vi "LV Test Semaphore 2.vi"() -> ()   [LabVIEW 2011]
panel:
  in  "milliseconds to wait":u32=500
  out "Wait Time":u32
  out "Hold Time":u32
  out "millisecond timer value 1":u32
  out "millisecond timer value 2":u32
  out "Locked 1":bool
  out "Numeric":i32
  out "Timed Out? 1":bool
  out "error out rel 2":errorcluster
  out "error out acq 2":errorcluster
  in  "Acq":bool
  in  "Open":bool
  in  "stop":bool
  out "Handle":u16
  out "error out create":errorcluster
  in  "Name":string="LabVIEW_System_Semaphore"
  out "error out destroy 1":errorcluster
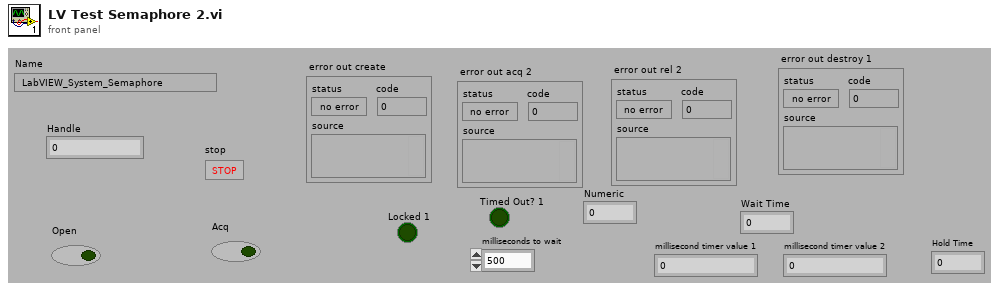
[diagram p1: front panel]
types:
  T1 = typedef "Semaphore RefNum" = refnum<k1>
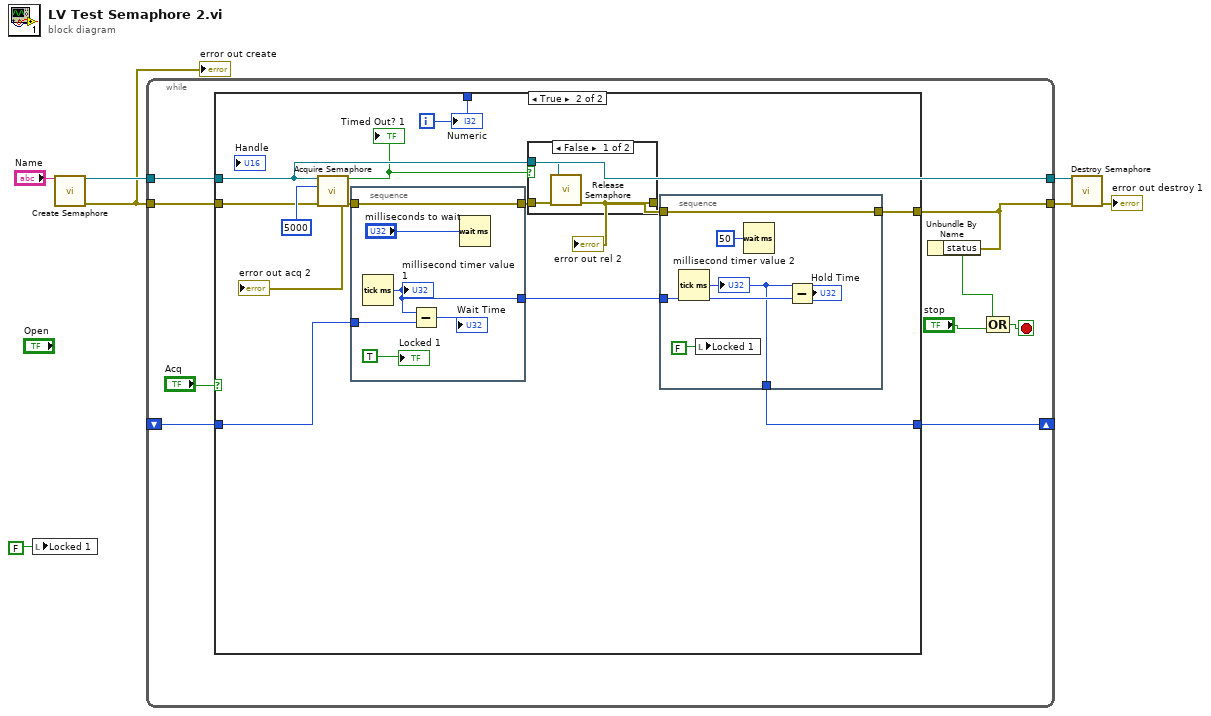
[diagram p0: block diagram]
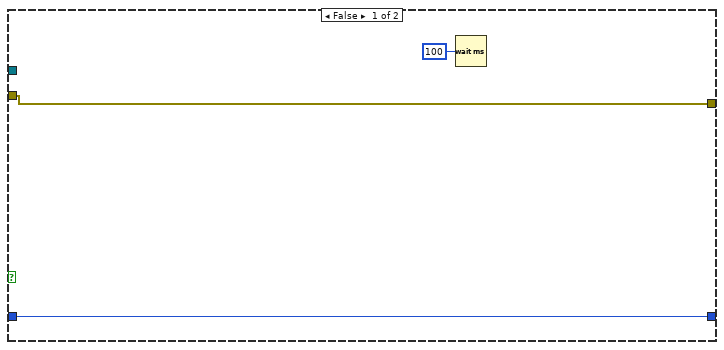
[diagram p2: hidden frame]
diagram:
  n1 = local write "Locked 1"(FALSE) -> ()
  n2 = call <vilib>:"Create Semaphore.vi"("name (unnamed)"="Name") -> ("error out"=w2:errorcluster, "semaphore"=w7:T1)  [unwired: 2 in, 3 out]
  "error out create" <- w2
  n3 = while {
    tunnel: w2 -> [w10]
    tunnel: w7 -> [w13]
    tunnel: [w13] -> w6
    tunnel: [w12] -> w5
    shift-right: [w9] -> _
    shift-left: _ -> [w8]
    i -> [w14]
    stop <- w16 stop-if-true
    n4 = case shown="True" "Acq" {
      tunnel: w14 -> [_ w32]
      tunnel: w13 -> [_ w26]
      tunnel: [w20 w30] -> w12
      tunnel: w10 -> [w20 w25]
      tunnel: [w18 w23] -> w9
      tunnel: w8 -> [w18 w22]
      frame False {
        n5 = Wait (ms)(milliseconds to wait=u32 100) -> ()  [unwired: 1 out]
      }
      frame True {
        n6 = call <vilib>:"Acquire Semaphore.vi"("error in (no error)"=w25, "ms timeout (-1)"=u16 5000 ("Timeout (ms)"), "semaphore"=w26) -> ("error out"=w29:errorcluster, "timed out"=w21:bool)  [unwired: 3 out]
        "Timed Out? 1" <- w21
        "error out acq 2" <- w29
        n7 = stacked-sequence {
          tunnel: w29 -> [w48]
          tunnel: [w48] -> w28
          tunnel: [w45] -> w24
          tunnel: w22 -> [w44]
          frame #0 {
            n8 = Tick Count (ms)() -> (millisecond timer value=w45:u32)
            "millisecond timer value 1" <- w45
            n9 = Subtract(x=w45, y=w44) -> (x-y=→"Wait Time":u32)
            n10 = Wait (ms)(milliseconds to wait="milliseconds to wait") -> ()  [unwired: 1 out]
            "Locked 1" <- TRUE
          }
        }
        n11 = case shown="False" w21 {
          tunnel: w28 -> [w35 w36]
          tunnel: w26 -> [w34 _]
          tunnel: [w33 w36] -> w27
          frame False {
            n12 = call <vilib>:"Release Semaphore.vi"("error in (no error)"=w35, "semaphore"=w34) -> ("error out"=w33:errorcluster)  [unwired: 5 out]
          }
          frame True {
          }
        }
        "error out rel 2" <- w27
        n13 = stacked-sequence {
          tunnel: w27 -> [w42]
          tunnel: [w42] -> w30
          tunnel: w24 -> [w39]
          tunnel: [w37] -> w23
          frame #0 {
            n14 = Tick Count (ms)() -> (millisecond timer value=w37:u32)
            "millisecond timer value 2" <- w37
            n15 = local write "Locked 1"(FALSE) -> ()
            n16 = Wait (ms)(milliseconds to wait=u32 50) -> ()  [unwired: 1 out]
            n17 = Subtract(x=w37, y=w39) -> (x-y=→"Hold Time":u32)
          }
        }
        "Numeric" <- w32
      }
    }
    n18 = Unbundle By Name(w12) -> ("status"=w15:bool)
    n19 = Compound Arithmetic op=OR(w15, "stop") -> (w16:bool)
  }
  n20 = call <vilib>:"Destroy Semaphore.vi"("error in (no error)"=w5, "semaphore"=w6) -> ("error out"=→"error out destroy 1":errorcluster)  [unwired: 5 out]
